vi "Multitone with Amplitudes and Phases.vi"() -> ()   [LabVIEW 2020]
doc: "Generates a multitone signal, then analyzes it for harmonic content."
uses:
  <vilib>/measure/matone.llb/Harmonic Distortion Analyzer.vi
  <vilib>/measure/NI_MAPro.lvlib
panel:
  out "components level":dbl[](array[numeric])
  out "detected fundamental frequency":dbl format="%#.6g"
  out "Spectrum":T1(graph)
  in  "amplitude 3":dbl=3.0 format="%#.6g"
  in  "amplitude 2":dbl=2.0 format="%#.6g"
  in  "amplitude 1":dbl=4.0 format="%#.6g"
  in  "phase 3":dbl=135.0 format="%#.6g"
  in  "phase 2":dbl=90.0 format="%#.6g"
  in  "phase 1":dbl format="%#.6g"
  in  "fundamental frequency":dbl=5.0
  in  "sampling info":cluster{"Fs":dbl, "#s":dbl}={"Fs"=100.0, "#s"=100.0} {"Fs" format="%#.6g"}
  out "Waveform":waveform(dbl)(graph)
  # "Overview: Generates a multitone signal, then analyzes it for harmonic content.\nRequirements: LabVIEW Full Development System\nInstructions:\nRun the VI."
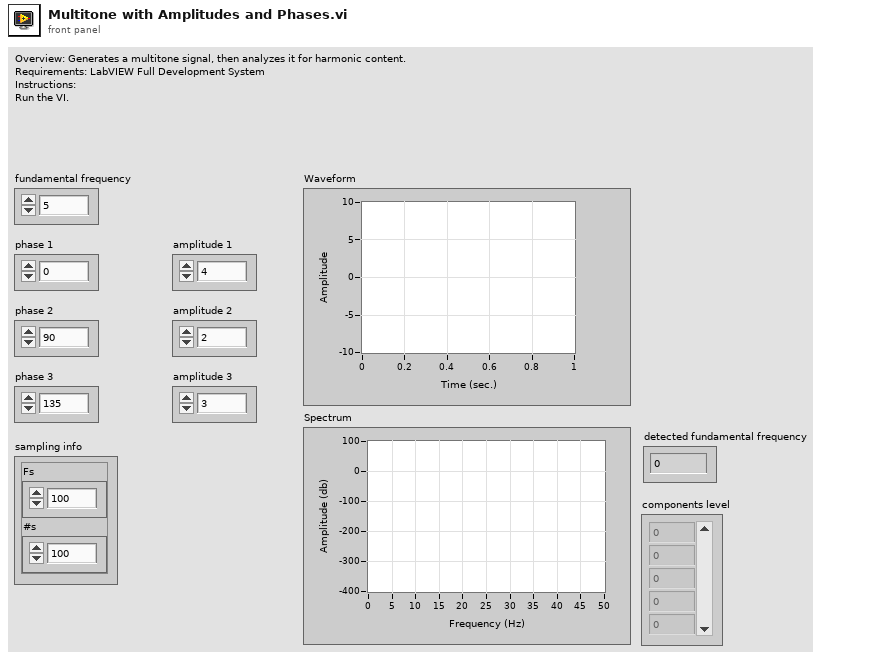
[diagram p1: front panel]
types:
  T1 = cluster{"f0":dbl, "df":dbl, "dB Spectrum (Hann)":dbl[]}
  T2 = enum16{"none", "input signal", "fundamental signal", "residual signal", "harmonics only", "noise and spurs"}
  T3 = cluster{"fundamental frequency":dbl, "search range %":dbl}
  T4 = cluster{"exported time signal":waveform(dbl), "exported spectrum (dB)":cluster{"f0":dbl, "df":dbl, "dB Spectrum (Hann)":dbl[]}}
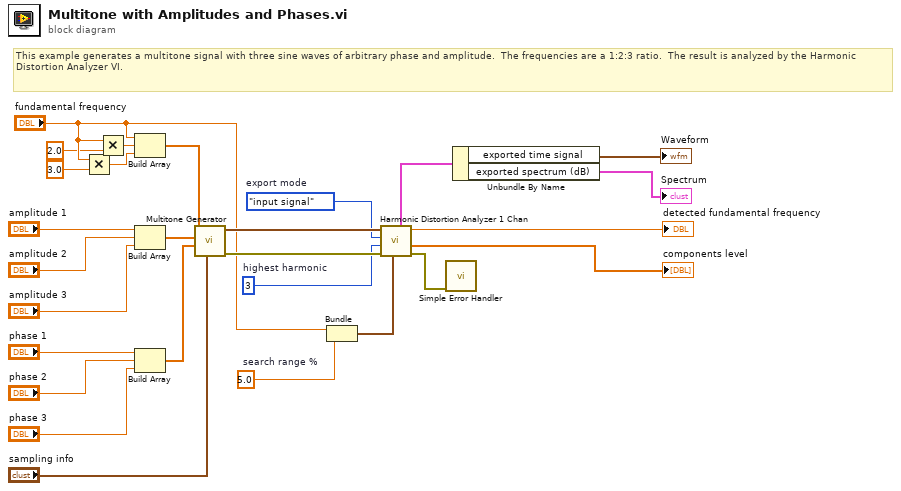
[diagram p0: block diagram]
diagram:
  w1 = 3  # highest harmonic
  w2 = 5.0  # search range %
  w7 = T2."input signal"  # export mode
  # "This example generates a multitone signal with three sine waves of arbitrary phase and amplitude.  The frequencies are a 1:2:3 ratio.  The result is analyzed by the Harmonic Distortion Analyzer VI."
  n1 = Multiply(x="fundamental frequency", y=3.0) -> (x*y=w13:dbl)
  n2 = Multiply(x="fundamental frequency", y=2.0) -> (x*y=w14:dbl)
  n3 = Build Array("fundamental frequency", w14, w13) -> (w10:dbl[])
  n4 = Build Array("amplitude 1", "amplitude 2", "amplitude 3") -> (w11:dbl[])
  n5 = Build Array("phase 1", "phase 2", "phase 3") -> (w12:dbl[])
  n6 = call <vilib>:"Multitone Generator.vi"("sampling info"="sampling info", "tone phases"=w12, "tone amplitudes"=w11, "tone frequencies"=w10) -> ("error out"=w25:errorcluster, "signal out"=w26:waveform(dbl))  [unwired: 4 in, 2 out]
  n7 = Bundle("fundamental frequency"="fundamental frequency", "search range %"=w2) -> (w9:T3)  [unwired: 1 in]
  n8 = call-poly <vilib>:"Harmonic Distortion Analyzer 1 Chan.vi"("advanced search"=w9, "error in (no error)"=w25, "highest harmonic"=w1, "export mode"=w7, "signal in"=w26) -> ("error out"=w5:errorcluster, "components level"=→"components level":dbl[], "detected fundamental frequency"=→"detected fundamental frequency":dbl, "exported signals"=w24:T4)  [unwired: 1 in, 2 out]
  n9 = call <vilib>:"Simple Error Handler.vi"("error in (no error)"=w5) -> ()  [unwired: 4 in, 5 out]
  n10 = Unbundle By Name(w24) -> ("exported time signal"=→"Waveform":waveform(dbl), "exported spectrum (dB)"=→"Spectrum":T1)
